vi "ReadDOs.vi"(8 "error in (no error)":errorcluster, 10 "Output":T1, 11 "VISA resource name":refnum<visa-resource-name>) -> (0 "error out":errorcluster, 2 "DOStatus":bool, 3 "VISA resource name out":refnum<visa-resource-name>)   [LabVIEW 2020, in "HandsOnPi2040.lvlib"]
uses:
  <instrlib>/HandsOnPi2040/HandsOnPi2040.lvlib
  <instrlib>/HandsOnPi2040/Public/DigOuts.ctl
  <instrlib>/HandsOnPi2040/cti-drivers-lv-visa-main/CTI-Visa/CTI-Visa.lvlib
panel:
  # "Output"
  # "Input"
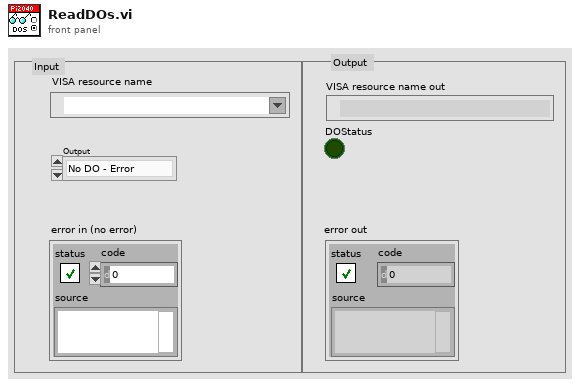
[diagram p1: front panel]
types:
  T1 = typedef "HandsOnPi2040.lvlib/DigOuts.ctl" = enum16{"No DO - Error", "DO1 (GPIO2)", "DO2 (GPIO3)", "DO3 (GPIO4)", "DO4 (GPIO5)", "BEEP (GPIO6)"}
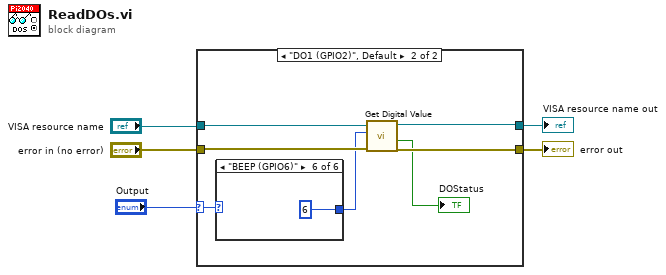
[diagram p0: block diagram]
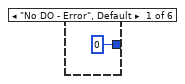
[diagram p3: hidden frame]
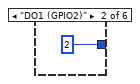
[diagram p4: hidden frame]
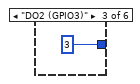
[diagram p5: hidden frame]
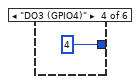
[diagram p6: hidden frame]
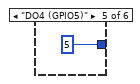
[diagram p7: hidden frame]
diagram:
  n1 = case shown="\"DO1 (GPIO2)\", Default" "Output" {
    selector: "Output" -> [_ w9]
    tunnel: "VISA resource name" -> [w7 w14]
    tunnel: [w7 w12] -> w5
    tunnel: [w6 w11] -> w4
    tunnel: "error in (no error)" -> [w6 w13]
    frame "No DO - Error" {
    }
    frame "DO1 (GPIO2)", Default {
      n2 = case shown="\"BEEP (GPIO6)\"" w9 {
        tunnel: [0 ("Channel") 2 ("Channel") 3 ("Channel") 4 ("Channel") 5 ("Channel") 6 ("Channel")] -> w8
        frame "No DO - Error", Default {
        }
        frame "DO1 (GPIO2)" {
        }
        frame "DO2 (GPIO3)" {
        }
        frame "DO3 (GPIO4)" {
        }
        frame "DO4 (GPIO5)" {
        }
        frame "BEEP (GPIO6)" {
        }
      }
      n3 = call <instrlib>:"Get Digital Value.vi"("error in (no error)"=w13, "Channel"=w8, "VISA resource name in"=w14) -> ("error out"=w11:errorcluster, "Value"=→"DOStatus":bool, "VISA resource name"=w12:refnum<visa-resource-name>)  [unwired: 6 in]
    }
  }
  "VISA resource name out" <- w5
  "error out" <- w4
